vi "Symphony Acquire Image.vi"(4 "Noise Substract":bool, 5 "Noise Mode":T1=enum."Selected Curve", 6 "AcqBusy":refnum<vi>, 7 "ImageMode":bool, 8 "error in":errorcluster caption="entrée d'erreur (pas d'erreur)", 9 "Accumulations":u16=1 min=1 step=1, 10 "ShutterEnable":bool, 11 "JYCCDLib.IJYCCDReqd":refnum<k7>) -> (0 "error out":errorcluster, 1 "Acq Time(ms)":u32, 2 "AcquisitionBusy":bool, 3 "Datas":i32[][][](array[numeric]))   [LabVIEW 2019]
uses:
  <userlib>/JY Symphony/NoiseCorr.ctl
  <userlib>/JY Symphony/Symphony Acq Image States.ctl
  <vilib>/Utility/error.llb/DialogType.ctl
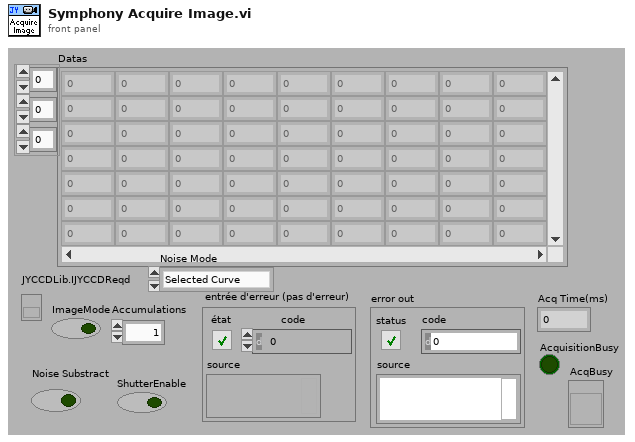
[diagram p1: front panel]
types:
  T1 = typedef "NoiseCorr.ctl" = enum16{"Off", "Selected Curve", "One For Every Acq"}
  T2 = typedef "Symphony Acq Image States.ctl" = enum16{"Start Acq", "Acq Busy", "ReqData", "GetDataObj", "AcqDone", "Error"}
  T3 = typedef "DialogType.ctl" = u16
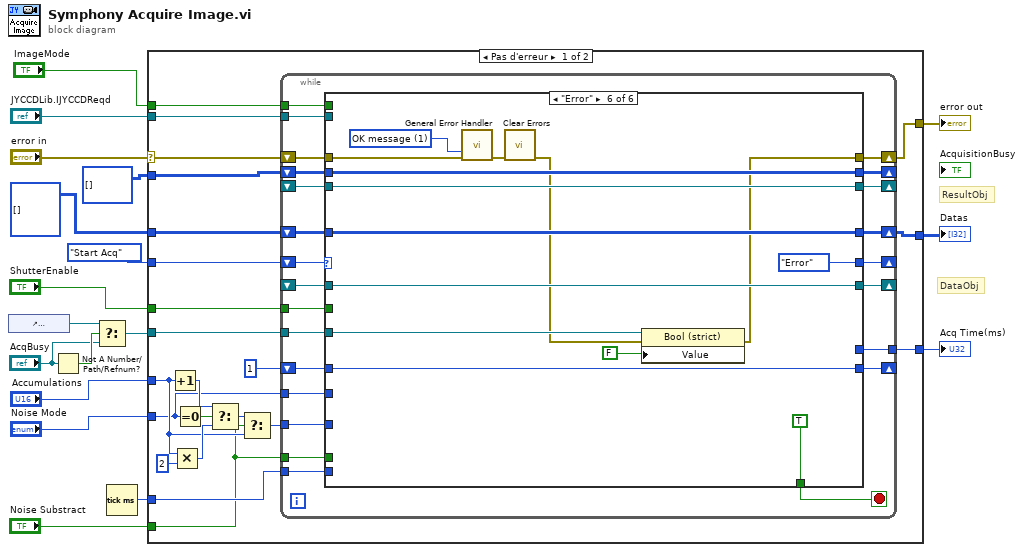
[diagram p0: block diagram]
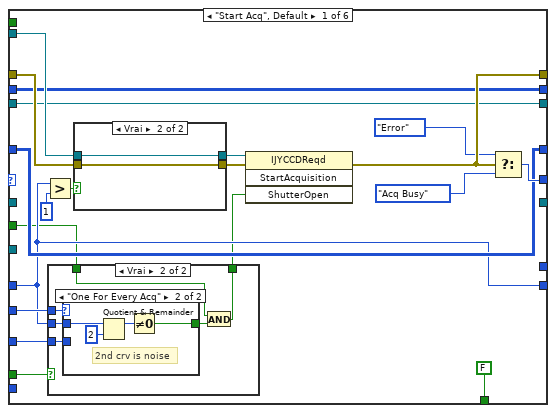
[diagram p2: hidden frame]
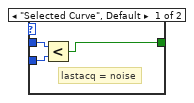
[diagram p4: hidden frame]
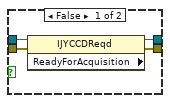
[diagram p5: hidden frame]
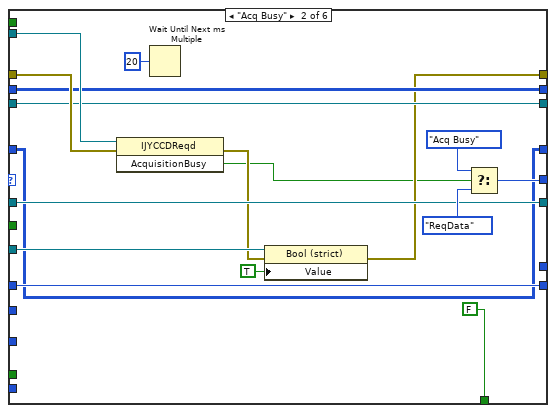
[diagram p6: hidden frame]
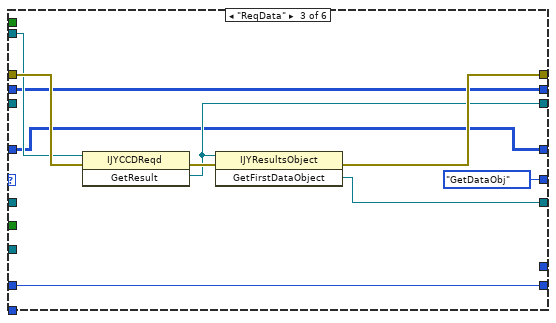
[diagram p7: hidden frame]
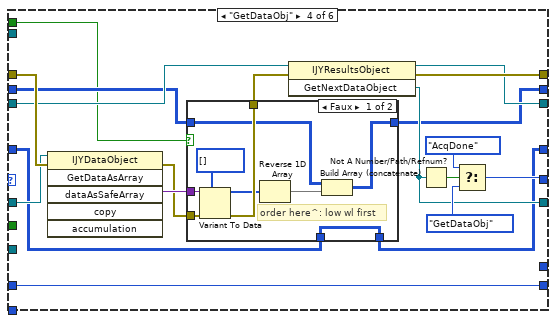
[diagram p8: hidden frame]
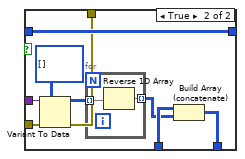
[diagram p9: hidden frame]
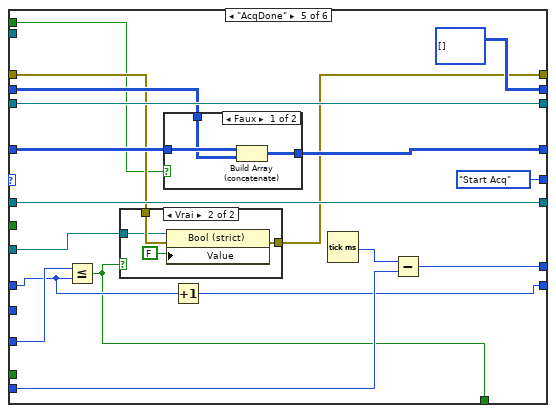
[diagram p10: hidden frame]
diagram:
  # "DataObj"
  # "ResultObj"
  n1 = control-ref of="AcquisitionBusy"() -> (w6:refnum<vi>)
  n2 = Not A Number/Path/Refnum?(number/path/refnum="AcqBusy") -> (NaN/Path/Refnum?=w7:bool)
  n3 = Select(t=w6, s=w7, f="AcqBusy") -> (s? t:f=w4:refnum<vi>)
  n4 = Tick Count (ms)() -> (millisecond timer value=w16:u32)
  n5 = case shown="Pas d'erreur" "error in" {
    selector: "error in" -> [w39 w212]
    tunnel: "JYCCDLib.IJYCCDReqd" -> [w40 _]
    tunnel: [w34 _] -> w18
    tunnel: w16 -> [w38 _]
    tunnel: Symphony_Acq_Image_States."Start Acq" -> [w37 _]
    tunnel: "ShutterEnable" -> [w36 _]
    tunnel: i32[][][] [] ("type") -> [w35 _]
    tunnel: [w33 _] -> w12
    tunnel: "Accumulations" -> [w23 _]
    tunnel: [w32 w212] -> w10
    tunnel: i32[][] [] ("type") -> [w31 _]
    tunnel: w4 -> [w30 _]
    tunnel: "ImageMode" -> [w29 _]
    tunnel: "Noise Substract" -> [w21 _]
    tunnel: "Noise Mode" -> [w19 _]
    frame No Error {
      n6 = Increment(x=w23) -> (x+1=w25:u16)
      n7 = Multiply(x=w23, y=u16 2) -> (x*y=w26:u16)
      n8 = Equal To 0?(x=w19) -> (x = 0?=w20:bool)
      n9 = Select(t=w25, s=w20, f=w26) -> (s? t:f=w24:u16)
      n10 = Select(t=w24, s=w21, f=w23) -> (s? t:f=w22:u16)
      n11 = while {
        tunnel: w40 -> [w61]
        tunnel: w38 -> [w63]
        shift-right: [w57] -> _
        shift-left: w37 -> [w62]
        shift-right: [w59] -> w32
        shift-left: w39 -> [w60]
        tunnel: w36 -> [w58]
        shift-right: [w56] -> _
        shift-left: _ -> [w52]
        shift-right: [w55] -> _
        shift-left: _ -> [w54]
        shift-right: [w64] -> w34
        shift-left: w35 -> [w53]
        tunnel: [w50] -> w33
        tunnel: w22 -> [w49]
        shift-right: [w47] -> _
        shift-left: u16 1 ("Accumulations:") -> [w48]
        shift-right: [w45] -> _
        shift-left: w31 -> [w46]
        tunnel: w30 -> [w44]
        tunnel: w29 -> [w43]
        tunnel: w21 -> [w42]
        tunnel: w19 -> [w41]
        stop <- w51 stop-if-true
        n12 = case shown="\"Error\"" w62 {
          tunnel: [w71 w106 w122 w132 w178 w210] -> w64
          tunnel: w63 -> [_ _ _ _ w187 _]
          tunnel: w61 -> [w82 w121 w129 _ _ _]
          tunnel: w60 -> [w81 w120 w131 w150 w174 w207]
          tunnel: [w80 w108 w128 w147 w173 w199] -> w59
          tunnel: w58 -> [w66 _ _ _ _ _]
          tunnel: [w77 w118 Symphony_Acq_Image_States."GetDataObj" w143 Symphony_Acq_Image_States."Start Acq" Symphony_Acq_Image_States."Error"] -> w57
          tunnel: [w73 w113 w127 w141 w181 w209] -> w56
          tunnel: [_ w112 w126 w140 w180 w208] -> w55
          tunnel: w54 -> [_ w112 _ w149 w180 w208]
          tunnel: w53 -> [w71 w106 w122 w133 w177 w210]
          tunnel: w52 -> [w73 w113 _ w148 w181 w209]
          tunnel: [FALSE FALSE _ _ w175 TRUE] -> w51
          tunnel: [_ _ _ _ w186 _] -> w50
          tunnel: w49 -> [w69 _ _ _ w184 _]
          tunnel: w48 -> [w68 w114 w124 w142 w183 w203]
          tunnel: [w68 w114 w124 w142 w182 w203] -> w47
          tunnel: w46 -> [w72 w111 w123 w138 w176 w202]
          tunnel: [w72 w111 w123 w139 i32[][] [] w202] -> w45
          tunnel: w44 -> [_ w110 _ _ w172 w201]
          tunnel: w43 -> [_ _ _ w134 w171 _]
          tunnel: w42 -> [w67 _ _ _ _ _]
          tunnel: w41 -> [w70 _ _ _ _ _]
          frame "Start Acq", Default {
            n13 = Greater?(x=w68, y=u16 1) -> (0:w75:bool)
            n14 = case shown="Vrai" w67 {
              tunnel: w70 -> [_ w91]
              tunnel: w69 -> [_ w90]
              tunnel: w68 -> [_ w89]
              tunnel: w66 -> [w85 w86]
              tunnel: [w85 w88] -> w65
              frame False {
              }
              frame True {
                n15 = case shown="\"One For Every Acq\"" w91 {
                  tunnel: w89 -> [w94 w98]
                  tunnel: w90 -> [w93 _]
                  tunnel: [w92 w95] -> w87
                  frame "Selected Curve", Default {
                    # "lastacq = noise"
                    n16 = Less?(x=w94, y=w93) -> (x < y?=w92:bool)
                  }
                  frame "One For Every Acq" {
                    # "2nd crv is noise"
                    n17 = Quotient & Remainder(x=w98, y=u16 2) -> (x-y*floor(x/y)=w96:u16)  [unwired: 1 out]
                    n18 = Not Equal To 0?(x=w96) -> (x != 0?=w95:bool)
                  }
                }
                n19 = And(x=w86, y=w87) -> (x .and. y?=w88:bool)
              }
            }
            n20 = case shown="Vrai" w75 {
              tunnel: [w102 w104] -> w84
              tunnel: [w101 w103] -> w83
              tunnel: w82 -> [w100 w104]
              tunnel: w81 -> [w99 w103]
              frame False {
                n21 = property class="IJYCCDReqd" props=["ReadyForAcquisition"](reference=w100, error in=w99) -> (reference out=w102:refnum<k7>, error out=w101:errorcluster)  [unwired: 1 out]
              }
              frame True {
              }
            }
            n22 = invoke class="IJYCCDReqd" method="StartAcquisition"(reference=w84, error in=w83, "ShutterOpen"=w65) -> (error out=w80:errorcluster)  [unwired: 1 in, 3 out]
            n23 = Select(t=Symphony_Acq_Image_States."Error", s=w80, f=Symphony_Acq_Image_States."Acq Busy") -> (s? t:f=w77:T2)
          }
          frame "Acq Busy" {
            n24 = invoke class="IJYCCDReqd" method="AcquisitionBusy"(reference=w121, error in=w120) -> (error out=w109:errorcluster, "AcquisitionBusy"=w107:bool)  [unwired: 1 in, 1 out]
            n25 = Wait Until Next ms Multiple(millisecond multiple=u32 20 ("n millisecondes")) -> ()  [unwired: 1 out]
            n26 = property class="Bool (strict)"(reference=w110, error in=w109, "Value"=TRUE ("Valeur")) -> (error out=w108:errorcluster)  [unwired: 1 out]
            n27 = Select(t=Symphony_Acq_Image_States."Acq Busy", s=w107, f=Symphony_Acq_Image_States."ReqData") -> (s? t:f=w118:T2)
          }
          frame "ReqData" {
            n28 = invoke class="IJYCCDReqd" method="GetResult"(reference=w129, error in=w131) -> (error out=w130:errorcluster, "GetResult"=w127:refnum<k7>)  [unwired: 1 in, 1 out]
            n29 = invoke class="IJYResultsObject" method="GetFirstDataObject"(reference=w127, error in=w130) -> (error out=w128:errorcluster, "GetFirstDataObject"=w126:refnum<k7>)  [unwired: 1 in, 1 out]
          }
          frame "GetDataObj" {
            n30 = invoke class="IJYDataObject" method="GetDataAsArray"(reference=w149, error in=w150) -> (error out=w136:errorcluster, "dataAsSafeArray"=w137:variant)  [unwired: 4 in, 4 out]
            n31 = case shown="Faux" w134 {
              tunnel: w138 -> [w154 w168]
              tunnel: [w159 w168] -> w139
              tunnel: w137 -> [w157 w167]
              tunnel: w136 -> [w156 w166]
              tunnel: [w155 w164] -> w135
              tunnel: w133 -> [w152 w163]
              tunnel: [w152 w162] -> w132
              frame False {
                # "order here^: low wl first"
                n32 = Variant To Data(error in=w156, type=i32[] [], Variant=w157) -> (data=w153:i32[], error out=w155:errorcluster)
                n33 = Reverse 1D Array(array=w153) -> (reversed array=w151:i32[])
                n34 = Build Array (concatenate)(w154, w151) -> (w159:i32[][])
              }
              frame True {
                n35 = Variant To Data(error in=w166, type=i32[][] [], Variant=w167) -> (data=w161:i32[][], error out=w164:errorcluster)
                n36 = for {
                  tunnel: w161 -> [w170] mode=indexing
                  tunnel: [w169] -> w160 mode=indexing
                  n37 = Reverse 1D Array(array=w170) -> (reversed array=w169:i32[])
                }
                n38 = Build Array (concatenate)(w163, w160) -> (w162:i32[][][])
              }
            }
            n39 = invoke class="IJYResultsObject" method="GetNextDataObject"(reference=w148, error in=w135) -> (reference out=w141:refnum<k7>, error out=w147:errorcluster, "GetNextDataObject"=w140:refnum<k7>)  [unwired: 1 in]
            n40 = Not A Number/Path/Refnum?(number/path/refnum=w140) -> (NaN/Path/Refnum?=w146:bool)
            n41 = Select(t=Symphony_Acq_Image_States."AcqDone", s=w146, f=Symphony_Acq_Image_States."GetDataObj") -> (s? t:f=w143:T2)
          }
          frame "AcqDone" {
            n42 = Less Or Equal?(x=w184, y=w183) -> (x <= y?=w175:bool)
            n43 = case shown="Vrai" w175 {
              tunnel: w174 -> [w193 w197]
              tunnel: [w193 w196] -> w173
              tunnel: w172 -> [_ w195]
              frame False {
              }
              frame True {
                n44 = property class="Bool (strict)"(reference=w195, error in=w197, "Value"=FALSE) -> (error out=w196:errorcluster)  [unwired: 1 out]
              }
            }
            n45 = case shown="Faux" w171 {
              tunnel: [w191 w192] -> w178
              tunnel: w177 -> [w190 w192]
              tunnel: w176 -> [w189 _]
              frame False {
                n46 = Build Array (concatenate)(w190, w189) -> (w191:i32[][][])
              }
              frame True {
              }
            }
            n47 = Increment(x=w183) -> (x+1=w182:u16)
            n48 = Tick Count (ms)() -> (millisecond timer value=w188:u32)
            n49 = Subtract(x=w188, y=w187) -> (x-y=w186:u32)
          }
          frame "Error" {
            w205 = T3 1 items=["no dialog", "OK message", "continue or stop message", "OK message + warnings", "continue/stop + warnings"] ("type of dialog (OK msg:1)")
            n50 = call <vilib>:"General Error Handler.vi"("type of dialog (OK msg:1)"=w205, "error in (no error)"=w207) -> ("error out"=w206:errorcluster)  [unwired: 9 in, 4 out]
            n51 = call <vilib>:"Clear Errors.vi"("error in (no error)"=w206) -> ("error out"=w200:errorcluster)  [unwired: 5 in, 1 out]
            n52 = property class="Bool (strict)"(reference=w201, error in=w200, "Value"=FALSE) -> (error out=w199:errorcluster)  [unwired: 1 out]
          }
        }
      }
    }
    frame Error {
    }
  }
  "Datas" <- w18
  "Acq Time(ms)" <- w12
  "error out" <- w10
